vi "upload.file_multipart_upload.vi"(8 "error in":errorcluster, 9 "timeout per chunk (ms)":i32=300000, 10 "File Path":path, 11 "Nominal Client in":refnum<class "Nominal Client.lvclass">) -> (0 "error out":errorcluster, 2 "S3 Path to File":string, 3 "Nominal Client out":refnum<class "Nominal Client.lvclass">)   [LabVIEW 2020, in "Nominal Client.lvclass"]
doc: "Handles the upload of files in a multipart format."
uses:
  Nominal Client.lvclass
  Nominal Client.lvclass/Nominal Client.ctl
  Nominal Client MultiPart Upload/Multipart Upload.lvclass
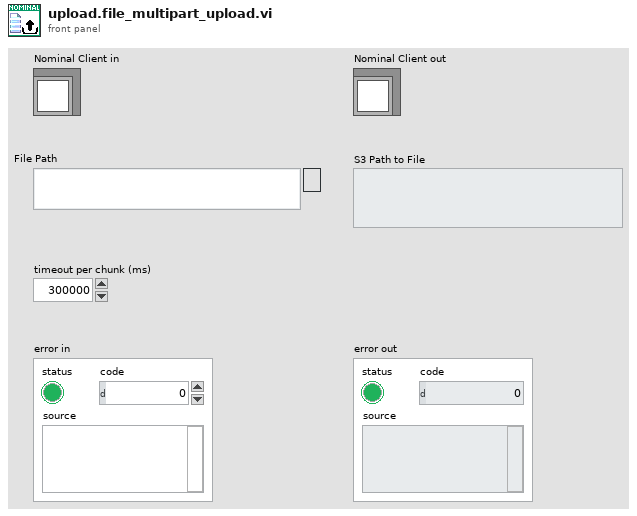
[diagram p1: front panel]
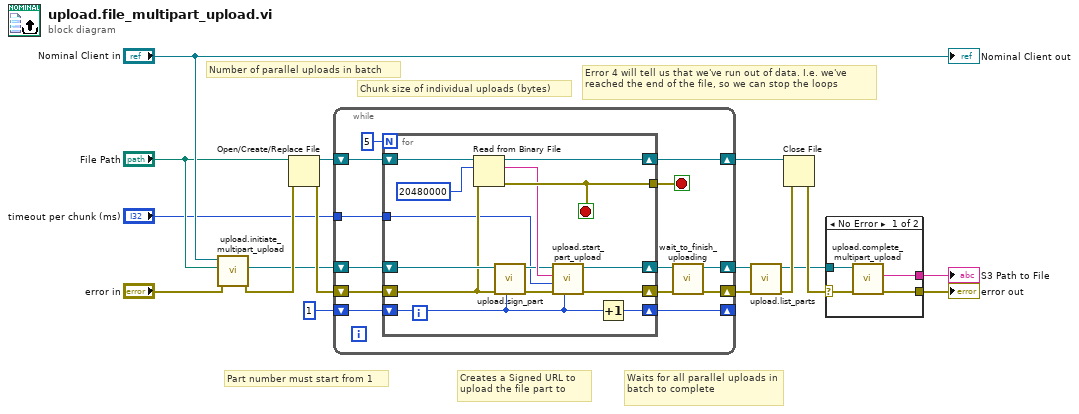
[diagram p0: block diagram]
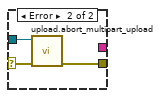
[diagram p2: hidden frame]
diagram:
  # "Waits for all parallel uploads in batch to complete"
  # "Creates a Signed URL to upload the file part to"
  # "Chunk size of individual uploads (bytes)"
  # "Number of parallel uploads in batch"
  # "Part number must start from 1"
  # "Error 4 will tell us that we've run out of data. I.e. we've reached the end of the file, so we can stop the loops"
  n1 = call "upload.initiate_multipart_upload.vi"("error in"="error in", "File Path"="File Path", "Nominal Client in"="Nominal Client in") -> ("error out"=w12:errorcluster, "Multipart Upload"=w10:refnum<class "Multipart Upload.lvclass">)  [unwired: 6 in, 1 out]
  n2 = Open/Create/Replace File(file path (use dialog)="File Path", error in=w12) -> (refnum out=w15:refnum<file>, error out=w11:errorcluster)  [unwired: 4 in, 1 out]
  n3 = while {
    shift-right: [w19] -> w17
    shift-left: w10 -> [w30]
    shift-right: [w22] -> w13
    shift-left: w11 -> [w24]
    shift-right: [w28] -> _
    shift-left: 1 -> [w29]
    shift-right: [w25] -> w14
    shift-left: w15 -> [w27]
    tunnel: "timeout per chunk (ms)" -> [w18]
    stop <- w26 stop-if-true
    n4 = for {
      N: 5 -> [_]
      shift-right: [w34] -> w20
      shift-left: w30 -> [w44]
      shift-right: [w43] -> w28
      shift-left: w29 -> [w33]
      tunnel: [w39] -> w26
      shift-right: [w40] -> w25
      shift-left: w27 -> [w41]
      shift-right: [w37] -> w23
      shift-left: w24 -> [w32]
      tunnel: w18 -> [w31]
      stop <- w39 stop-if-true
      n5 = Read from Binary File(8:w32, 10:20480000 ("count (1)"), 11:w41) -> (0:w39:errorcluster, 2:w36:string, 3:w40:refnum<file>)  [unwired: 3 in, 1 out]
      n6 = call "upload.sign_part.vi"("Part Number"=w33, "error in"=w32, "Multipart Upload in"=w44) -> ("error out"=w38:errorcluster, "Multipart Upload out"=w35:refnum<class "Multipart Upload.lvclass">)  [unwired: 7 in]
      n7 = call "upload.start_part_upload.vi"("Part Number"=w33, "error in"=w38, "timeout (ms)"=w31, "File Part Binary"=w36, "Multipart Upload"=w35) -> ("error out"=w37:errorcluster, "Multipart Upload out"=w34:refnum<class "Multipart Upload.lvclass">)  [unwired: 5 in]
      n8 = Increment(x=w33) -> (x+1=w43:i32)
    }
    n9 = call "wait_to_finish_uploading.vi"("error in"=w23, "Multipart Upload in"=w20) -> ("error out"=w22:errorcluster, "Multipart Upload out"=w19:refnum<class "Multipart Upload.lvclass">)  [unwired: 8 in]
  }
  n10 = call "upload.list_parts.vi"("error in"=w13, "Multipart Upload"=w17) -> ("error out"=w9:errorcluster, "Multipart Upload out"=w7:refnum<class "Multipart Upload.lvclass">)  [unwired: 8 in]
  n11 = Close File(refnum=w14, error in=w9) -> (error out=w8:errorcluster)  [unwired: 1 out]
  n12 = case shown="No Error" w8 {
    selector: w8 -> [w46 w51]
    tunnel: [w48 _] -> w6
    tunnel: w7 -> [w47 w50]
    tunnel: [w45 w49] -> w5
    frame No Error {
      n13 = call "upload.complete_multipart_upload.vi"("error in"=w46, "Multipart Upload in"=w47) -> ("error out"=w45:errorcluster, "S3 Path to File"=w48:string)  [unwired: 8 in]
    }
    frame Error {
      n14 = call "upload.abort_multipart_upload.vi"("error in"=w51, "Multipart Upload"=w50) -> ("error out"=w49:errorcluster)  [unwired: 9 in]
    }
  }
  "error out" <- w5
  "S3 Path to File" <- w6
  "Nominal Client out" <- "Nominal Client in"
